vi "Vector2DArrayNormalize.vi"(11 "Vector Array":T1[](array[typedef])) -> (3 "Normalized Vector Array":T1[](array[typedef]))   [LabVIEW 2018]
uses:
  Vector2D.ctl
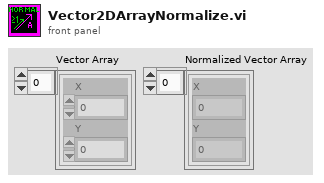
[diagram p1: front panel]
types:
  T1 = typedef "Vector2D.ctl" = cluster{"X":dbl, "Y":dbl}
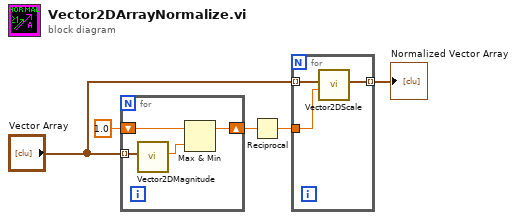
[diagram p0: block diagram]
diagram:
  n1 = for {
    tunnel: "Vector Array" -> [w9] mode=indexing
    shift-right: [w8] -> w4
    shift-left: 1.0 -> [w7]
    n2 = call "Vector2DMagnitude.vi"("Vector"=w9) -> ("Magnitude"=w6:dbl)  [unwired: 10 in]
    n3 = Max & Min(x=w7, y=w6) -> (max(x,y)=w8:dbl)  [unwired: 1 out]
  }
  n4 = Reciprocal(x=w4) -> (1/x=w2:dbl)
  n5 = for {
    tunnel: "Vector Array" -> [w12] mode=indexing
    tunnel: w2 -> [w11]
    tunnel: [w10] -> w1 mode=indexing
    n6 = call "Vector2DScale.vi"("Scale Factor"=w11, "Vector"=w12) -> ("Scaled Vector"=w10:T1)  [unwired: 9 in]
  }
  "Normalized Vector Array" <- w1
